vi "Wave1D_Solve AU.vi"(9 "LU of A":T1, 10 "A":T3, 11 "U":dbl[](array[numeric])) -> (0 "error":i32, 3 "A\\U":dbl[](array[numeric]))   [LabVIEW 2020, in "NI_PDE.lvlib"]
uses:
  <vilib>/gmath/NI_PDE.lvlib
  <vilib>/Analysis/Matrix/Datatypes/RealMatrix.ctl
  <vilib>/Analysis/7linalg.llb/Solve Linear Equations (single right hand).vi
  <vilib>/Analysis/baseanly.llb/Solve Linear Equations By Cholesky.vi
  <vilib>/Analysis/baseanly.llb/Real Matrix to Compact Array.vi
  <vilib>/Analysis/baseanly.llb/Real Compact Tri-Matrix Linear Eqs.vi
  <vilib>/Analysis/7linalg.llb/Solve Linear Eqs (General).vi
  <vilib>/Analysis/7linalg.llb/Solve Linear Eqs (Gen, single right hand).vi
  <vilib>/Analysis/NI_AALPro.lvlib
  <vilib>/Analysis/Matrix/NI_Matrix.lvlib
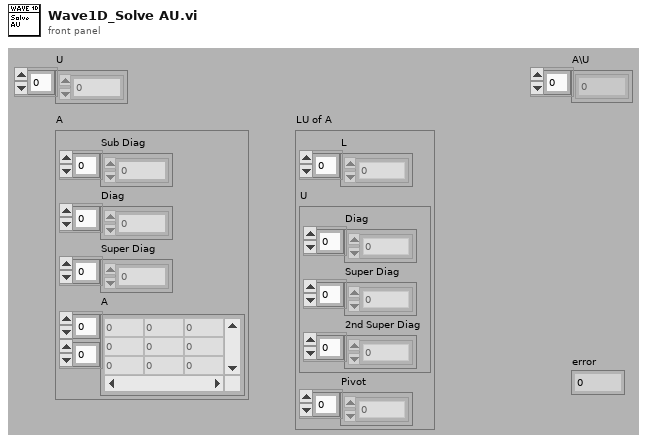
[diagram p1: front panel]
types:
  T1 = cluster{"L":dbl[], "U":cluster{"Diag":dbl[], "Super Diag":dbl[], "2nd Super Diag":dbl[]}, "Pivot":i32[]}
  T2 = typedef "NI_Matrix.lvlib/RealMatrix.ctl" = dbl[][]
  T3 = cluster{"Sub Diag":dbl[], "Diag":dbl[], "Super Diag":dbl[], "A":T2}
  T4 = cluster{"Diag":dbl[], "Super Diag":dbl[], "2nd Super Diag":dbl[]}
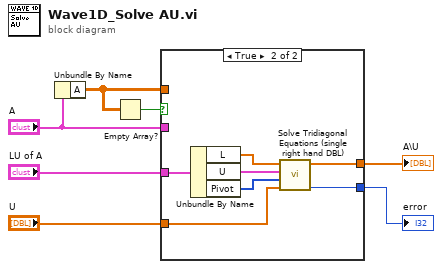
[diagram p0: block diagram]
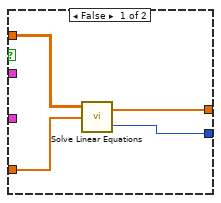
[diagram p2: hidden frame]
diagram:
  n1 = Unbundle By Name("A") -> ("A"=w5:T2)
  n2 = Empty Array?(array=w5) -> (empty?=w7:bool)
  n3 = case shown="True" w7 {
    tunnel: "U" -> [w10 w14]
    tunnel: w5 -> [w11 _]
    tunnel: [w9 w13] -> w4
    tunnel: [w8 w12] -> w2
    tunnel: "A" -> [_ _]
    tunnel: "LU of A" -> [_ w18]
    frame False {
      n4 = call-poly <vilib>:"Solve Linear Equations.vi"("Known Vector"=w10, "Input Matrix"=w11) -> ("error"=w8:i32, "Solution Vector"=w9:dbl[])  [unwired: 1 in]
    }
    frame True {
      n5 = Unbundle By Name(w18) -> ("L"=w17:dbl[], "U"=w16:T4, "Pivot"=w15:i32[])
      n6 = call <vilib>:"Solve Tridiagonal Equations (single right hand DBL).vi"("Known Vector"=w14, "Pivot"=w15, "U"=w16, "L"=w17) -> ("error"=w12:i32, "Solution Vector"=w13:dbl[])  [unwired: 6 out]
    }
  }
  "A\\U" <- w4
  "error" <- w2
